vi "FGVTimer.vi"(10 "set timer":dbl=-1.0, 11 "Reset":bool) -> (2 "Elapsed?":bool, 3 "Time Elapsed":dbl)   [LabVIEW 2019]
doc: "Timer semplice che si basa su un numero random come limite di tempo massimo"
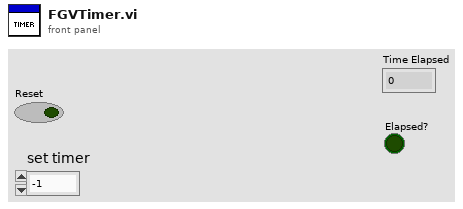
[diagram p1: front panel]
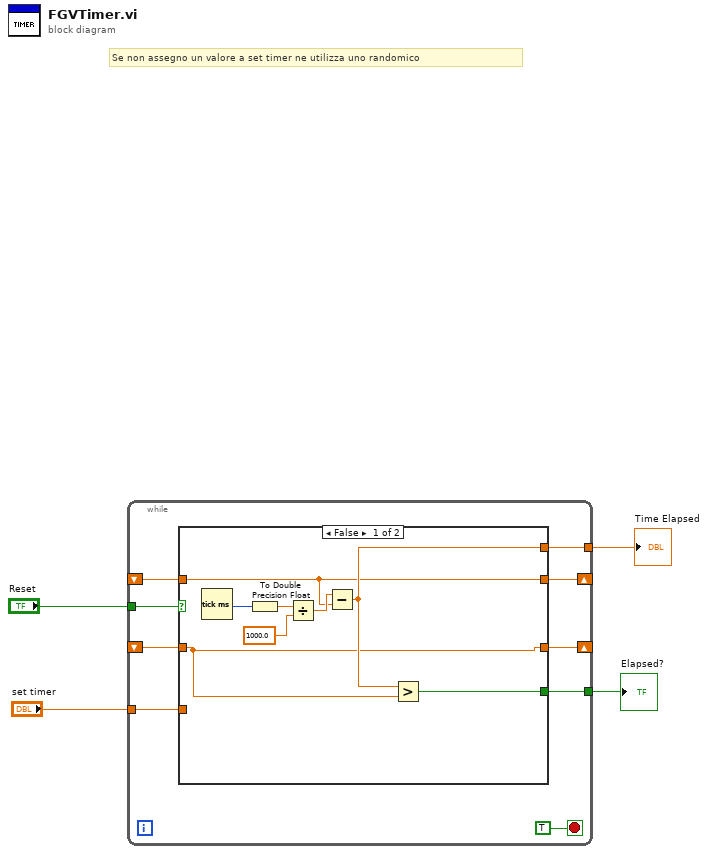
[diagram p0: block diagram]
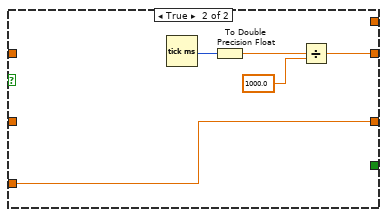
[diagram p2: hidden frame]
diagram:
  # "Se non assegno un valore a set timer ne utilizza uno randomico"
  n1 = while {
    tunnel: "set timer" -> [w10]
    tunnel: "Reset" -> [w12]
    shift-right: [w11] -> _
    shift-left: _ -> [w8]
    shift-right: [w9] -> _
    shift-left: _ -> [w7]
    tunnel: [w6] -> w2
    tunnel: [w5] -> w1
    stop <- TRUE stop-if-true
    n2 = case shown="False" w12 {
      tunnel: [w14 w23] -> w11
      tunnel: w10 -> [_ w25]
      tunnel: [w16 w25] -> w9
      tunnel: w8 -> [w14 _]
      tunnel: w7 -> [w16 _]
      tunnel: [w18 _] -> w6
      tunnel: [w17 _] -> w5
      frame False {
        n3 = Tick Count (ms)() -> (millisecond timer value=w21:u32)
        n4 = To Double Precision Float(number=w21) -> (double precision float=w20:dbl)
        n5 = Divide(x=w20, y=1000.0) -> (x/y=w15:dbl)
        n6 = Subtract(x=w15, y=w14) -> (x-y=w17:dbl)
        n7 = Greater?(x=w17, y=w16) -> (0:w18:bool)
      }
      frame True {
        n8 = Tick Count (ms)() -> (millisecond timer value=w26:u32)
        n9 = To Double Precision Float(number=w26) -> (double precision float=w24:dbl)
        n10 = Divide(x=w24, y=1000.0) -> (x/y=w23:dbl)
      }
    }
  }
  "Time Elapsed" <- w1
  "Elapsed?" <- w2
